vi "Cure.vi"(8 "Error In":errorcluster, 11 "Selection List[]":refnum<vi>[](array[refnum])) -> (0 "Error Out":errorcluster, 3 "Change Made?":bool)   [LabVIEW 2017, in "Eulogy.lvlib"]
doc: "Changes a grave site (Diagram Disable structure) to the Spirit frame (refactored code) and enables it. In other words, cure the zombie infection that has occurred within the block diagram. This is the opposite of infecting a corpse."
uses:
  Eulogy.lvlib
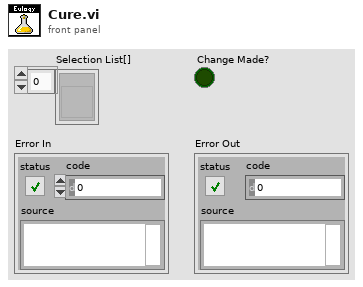
[diagram p1: front panel]
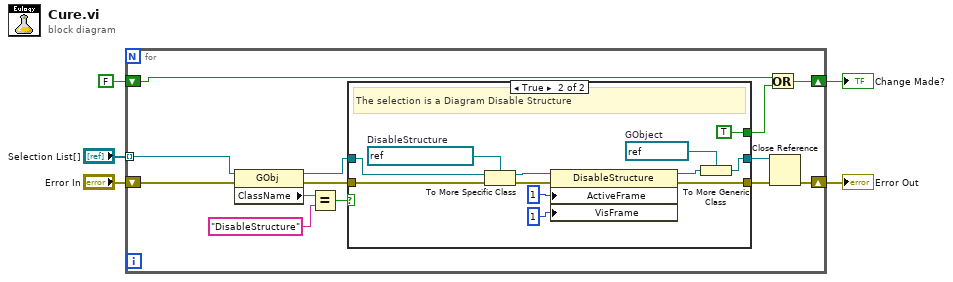
[diagram p0: block diagram]
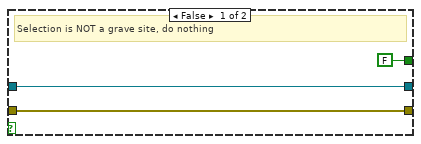
[diagram p2: hidden frame]
diagram:
  n1 = for {
    shift-right: [w6] -> w5
    shift-left: "Error In" -> [w18]
    tunnel: "Selection List[]" -> [w12] mode=indexing
    shift-right: [w9] -> w3
    shift-left: FALSE -> [w11]
    n2 = property class="GObj"(reference=w12, error in=w18) -> (reference out=w14:refnum<vi>, error out=w13:errorcluster, "ClassName"=w17:string)
    n3 = Equal?(x=w17, y="DisableStructure") -> (x = y?=w15:bool)
    n4 = case shown="True" w15 {
      tunnel: w14 -> [w20 w32]
      tunnel: w13 -> [w19 w31]
      tunnel: [FALSE ("y") TRUE ("y")] -> w10
      tunnel: [w19 w25] -> w8
      tunnel: [w20 w23] -> w7
      frame False {
        # "Selection is NOT a grave site, do nothing"
      }
      frame True {
        w22 = refnum<vi> refnum  # GObject
        w33 = refnum<vi> refnum  # DisableStructure
        # "The selection is a Diagram Disable Structure"
        n5 = To More Specific Class(target class=w33, reference=w32, error in=w31) -> (specific class reference=w29:refnum<vi>, error out=w30:errorcluster)
        n6 = property class="DisableStructure"(reference=w29, error in=w30, "ActiveFrame"=i16 1 ("Active Frame"), "VisFrame"=u32 1 ("Visible Frame")) -> (reference out=w26:refnum<vi>, error out=w25:errorcluster)
        n7 = To More Generic Class(target class=w22, reference=w26) -> (generic class reference=w23:refnum<vi>)
      }
    }
    n8 = Or(x=w11, y=w10) -> (x .or. y?=w9:bool)
    n9 = Close Reference(reference=w7, error in (no error)=w8) -> (error out=w6:errorcluster)
  }
  "Error Out" <- w5
  "Change Made?" <- w3
